vi "Dashboard Main.vi"() -> ()   [LabVIEW 2012]
uses:
  <vilib>/event_ctls.llb/eventvkey.ctl
  <vilib>/Utility/config.llb/Read Key (String).vi
  <vilib>/Utility/config.llb/Read Key (I32).vi
  <vilib>/Utility/config.llb/Write Key (String).vi
  <vilib>/Utility/config.llb/Write Key (I32).vi
  <vilib>/Utility/config.llb/NI_LVConfig.lvlib
  <vilib>/vision/NI_Vision_Development_Module.lvlib
panel:
  out "Battery Value":dbl(slide) scale=0.0..14.0 scale format="%#_2e"
  out "Battery":sgl(graph)
  in  "Camera Settings":T1={"Frate Rate"=30, "Compression"=30, "Size"=1} {"Frate Rate" scale=1.0..30.0; "Size" items=["640x480", "320x240", "160x120"]}
  out "Mode":T2(ring)=enum."Auto Disabled"
  out "Camera IP":string
  out "JS1 Z":dbl(slide) scale=-1.0..1.0 scale format="%#_2e"
  out "JS2 Z":dbl(slide) scale=-1.0..1.0 scale format="%#_2e"
  out "Joystick 1":cluster{"X":dbl, "Y":dbl}[](graph)
  out "Joystick 2":cluster{"X":dbl, "Y":dbl}[](graph)
  out "JS Buttons 1":T3
  out "JS Buttons 2":T3
  out "MotorSlide4":dbl(slide) scale=-1.0..1.0 scale format="%#_2e"
  out "MotorSlide3":dbl(slide) scale=-1.0..1.0 scale format="%#_2e"
  out "MotorSlide2":dbl(slide) scale=-1.0..1.0 scale format="%#_2e"
  in  "MotorName3":string="Front Left"
  in  "MotorName4":string="Front Right"
  in  "MotorName1":string="Rear Left"
  in  "MotorName2":string="Rear Right"
  out "MotorChart4":dbl(graph)
  out "MotorChart3":dbl(graph)
  out "MotorChart2":dbl(graph)
  out "MotorSlide1":dbl(slide) scale=-1.0..1.0 scale format="%#_2e"
  out "MotorChart1":dbl(graph)
  out "Robot IP":string
  in  "Dashboard Tab":enum32{"Operation", "Test", "Checklist"}(tab)
  in  "Checkbox 2":bool
  in  "Checkbox 1":bool
  in  "Slider 1":dbl(slide) scale=0.0..100.0
  out "Target Center":dbl[](array[numeric])
  in  "Slider":dbl(slide) scale=0.0..100.0 scale format="%#_3g"
  in  "On/Off":bool caption="Solenoid"
  in  "Test Name":u16(ring) items=["Select the test to run...", "Example Test", "-------------------------------", "List of tests is built in robot code.", "Replace with your own automated tests."]
  in  "Test Tree":string(tree)
  in  "Motor":cluster{"Value":dbl, "Enable":bool} {"Value" scale=-1.0..1.0 scale format="%#_3g"}
  out "Progress":T4 {"Test Progress" scale=0.0..100.0}
  in  "Rev/Fwd":cluster{"Forward":bool, "Reverse":bool}
  in  "Ring":u16(ring) items=["Auto", "Fixed indoor", "Fixed outdoor 1", "Fixed outdoor 2", "Fixed fluorescent 1", "Fixed fluorescent 2", "Hold current"]
  in  "Listbox":i32(listbox)
  in  "Viewer":T5(tab)
  out "Mbps":dbl format="%#.1g"
  in  "Enable":bool
  in  "DB Camera Config":bool
  out "Mbps":bool
  out "fps":dbl format="%#.1g"
  out "Image Error Message":string="Timeout in Camera Communications"
  out "Camera Image":T6(plugin-control)
  out "Buttons 1":cluster{"1":bool, "2":bool, "3":bool}
  out "Kinect 1":cluster{"X":dbl, "Y":dbl, "Z":dbl} {"X" scale=1.0..-1.0; "Y" scale=1.0..-1.0; "Z" scale=1.0..-1.0}
  out "Buttons 2":cluster{"1":bool, "2":bool, "3":bool}
  out "Kinect 2":cluster{"X":dbl, "Y":dbl, "Z":dbl} {"X" scale=1.0..-1.0; "Y" scale=1.0..-1.0; "Z" scale=1.0..-1.0}
  out "Version":string
  out "Skeleton Picture":picture
  out "Players":i8
  out "Tree":string(tree)
  out "Camera Image 2":T6(plugin-control)
  in  "Hue Range":cluster{dbl, dbl}
  in  "Sat Range":cluster{dbl, dbl}
  in  "Lum Range":cluster{dbl, dbl}
  # "Drive & Motors"
  # "Robot IP:"
  # "Customize by placing controls and indicators here and name to match\nDashboard Variables on robot."
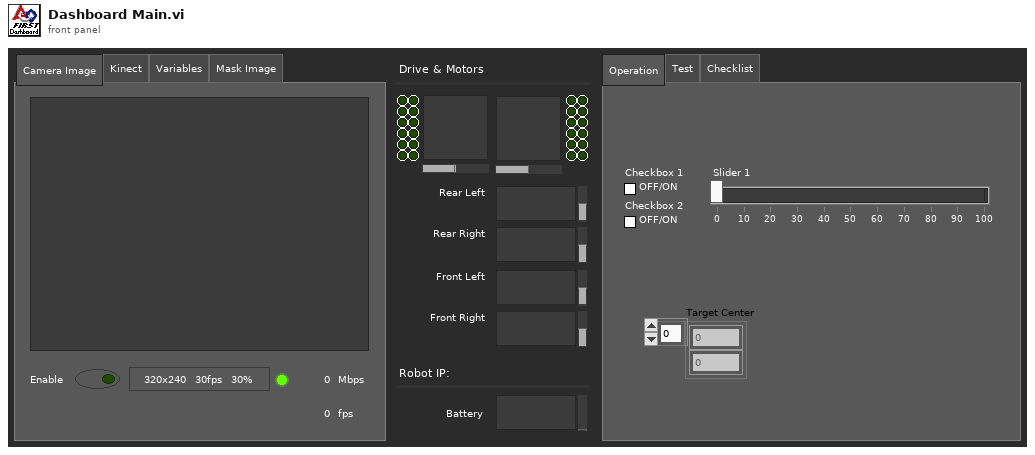
[diagram p1: front panel]
types:
  T1 = cluster{"Frate Rate":i32, "Compression":i32, "Size":u16}
  T2 = enum8{"Tele-Op Disabled", "Tele-Op Enabled", "Auto Disabled", "Auto Enabled", "Test Disabled", "Test Enabled", ""}
  T3 = cluster{bool, bool, bool, bool, bool, bool, bool, bool, bool, bool, bool, bool}
  T4 = cluster{"Test Progress":u8, "Test Progress Text":string}
  T5 = enum32{"Camera Image", "Kinect", "Variables", "Mask Image"}
  T6 = typedef "IMAQ Image.ctl" = refnum<image>
  T7 = typedef "Image Type" = u32
  T8 = typedef "LVBoundsTypeDef.ctl" = cluster{"Width":u32, "Height":u32}
  T9 = typedef "SkeletonTrackState.ctl" = enum32{"NotTracked", "PositionOnly", "Tracked"}
  T10 = cluster{"TrackingState":u8[], "Position":cluster{"x":sgl, "y":sgl, "z":sgl}, cluster{"x":sgl, "y":sgl, "z":sgl, sgl}[], "TrackState":T9}
  T11 = cluster{cluster{"ScaledToPercentRange":dbl, "ScaledToPercentRange":dbl, "ScaledToPercentRange":dbl}, cluster{bool, bool, bool}}[]
  T12 = cluster{cluster{"ScaledToPercentRange":dbl, "ScaledToPercentRange":dbl, "ScaledToPercentRange":dbl}, cluster{bool, bool, bool}}
  T13 = cluster{"ScaledToPercentRange":dbl, "ScaledToPercentRange":dbl, "ScaledToPercentRange":dbl}
  T14 = typedef "LVRectTypeDef.ctl" = cluster{"Left":i16, "Top":i16, "Right":i16, "Bottom":i16}
  T15 = cluster{"Competition mode":bool, "Robot Link":bool, "Autonomous":bool, "Enabled":bool, "E-Stop":bool, "Simulated":bool, "TestMode":bool, "Docked Window":bool}
  T16 = cluster{"Boolean Array[0]":bool, "Boolean Array[1]":bool, "Boolean Array[2]":bool, "Boolean Array[3]":bool, "Boolean Array[4]":bool, "Boolean Array[5]":bool, "Boolean Array[6]":bool, "Boolean Array[7]":bool, "Boolean Array[8]":bool, "Boolean Array[9]":bool, "Boolean Array[10]":bool, "Boolean Array[11]":bool}
  T17 = cluster{"Position":cluster{"X":dbl, "Y":dbl}, "Distance (ft)":dbl, "Center":bool}[]
  T18 = cluster{"Rect Coverage":i32, "X Edge Strength":i32, "Y Edge Strength":i32, "Center":i32, "Outer":i32}
  T19 = cluster{cluster{"Left":dbl, "Top":dbl, "Right":dbl, "Bottom":dbl}, "Scores":dbl[], cluster{"Long":dbl, "Short":dbl}}[]
  T20 = cluster{"Target Center (-1 to 1)":cluster{"X":dbl, "Y":dbl}, "Distance (ft)":dbl, "Center Target":bool}
  T21 = cluster{"Target Center (-1 to 1)":cluster{"X":dbl, "Y":dbl}, "Distance (ft)":dbl, "Center Target":bool}[]
  T22 = cluster{"Left":dbl, "Top":dbl, "Right":dbl, "Bottom":dbl}
  T23 = typedef "NI_LVConfig.lvlib/Config Data RefNum.ctl" = refnum<k1>
  T24 = typedef "eventvkey.ctl" = enum16{"ASCII", "Enter", "Return", "Shift", "Ctrl", "Alt", "Cmd", "Opt", "Caps", "NumLock", "Clear", "Break", "Up", "Down", "Left", "Right", "Insert", "Delete", "Home", "End", "PageUp", "PageDown", "Escape", "Help", "Pause", "ScrollLock", "F1", "F2", "F3", "F4", "F5", "F6", "F7", "F8", "F9", "F10", "F11", "F12", "F13", "F14", "F15", "F16", "F17", "F18", "F19", "F20", "F21", "F22", "F23", "F24", "Play", "VolumeUp", "VolumeDown", "Mute", "Two Byte Char"}
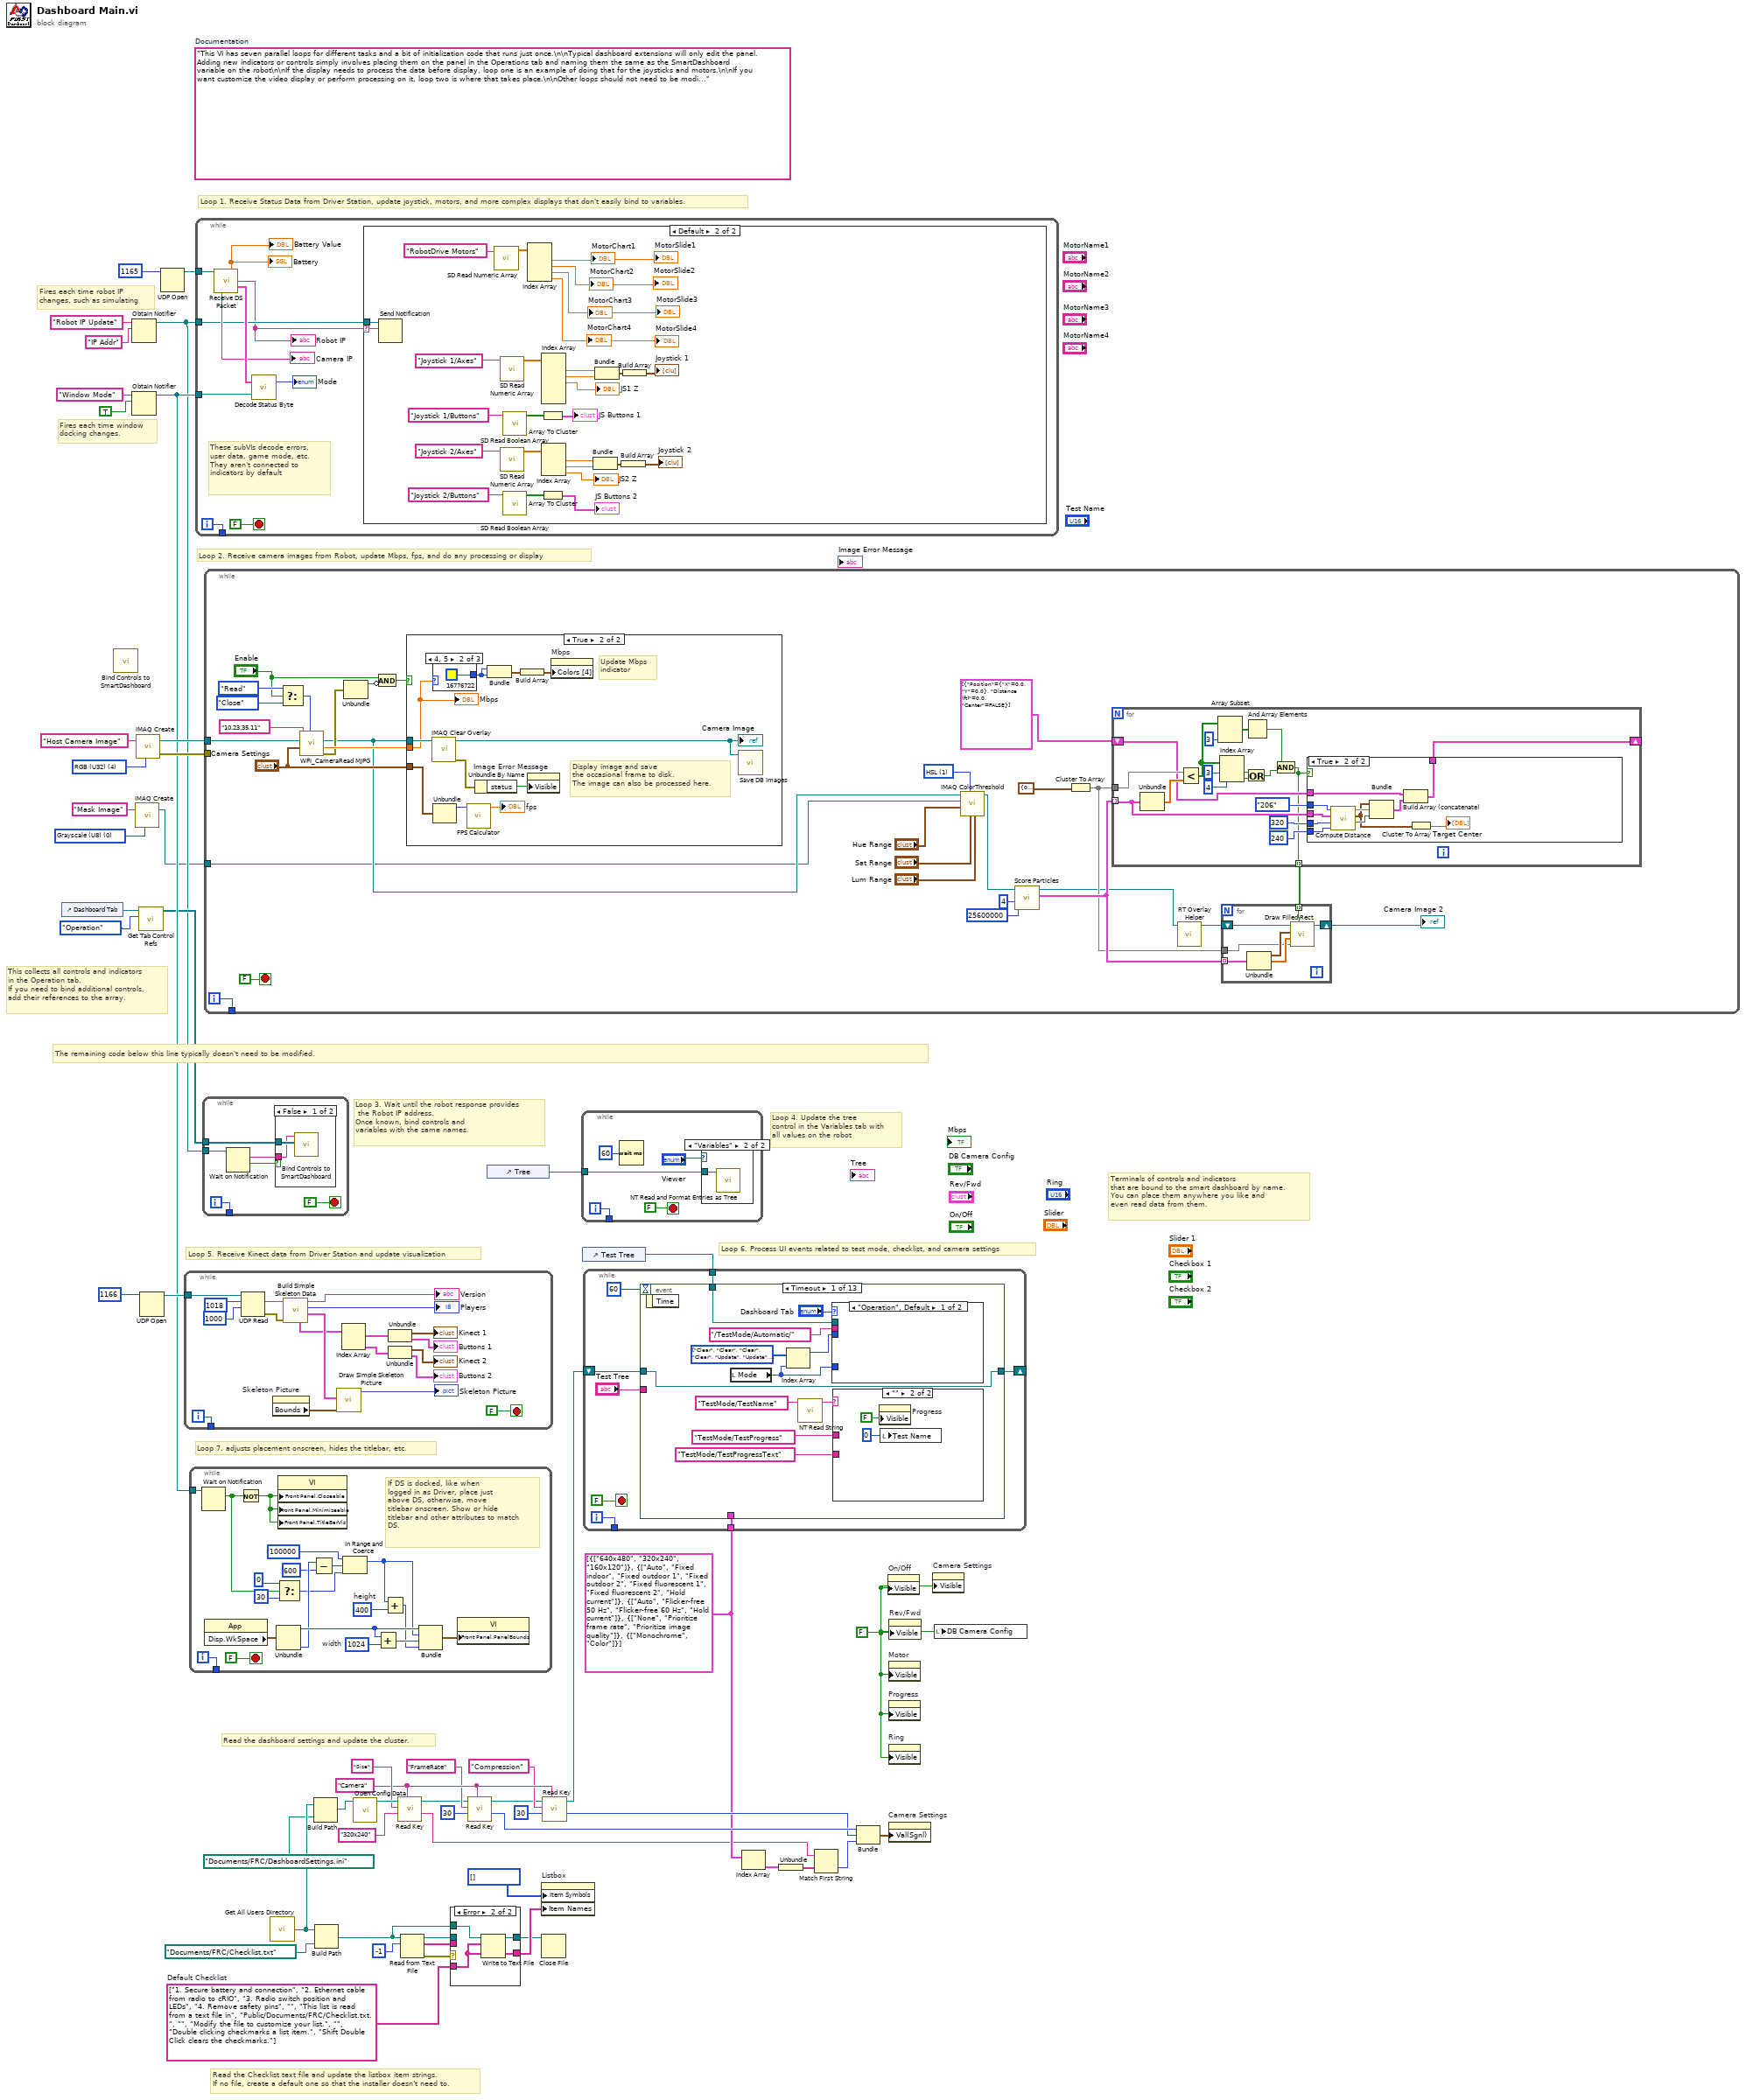
[diagram p0: block diagram]
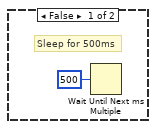
[diagram p4: hidden frame]
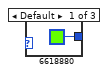
[diagram p5: hidden frame]
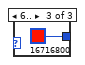
[diagram p6: hidden frame]
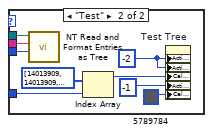
[diagram p8: hidden frame]
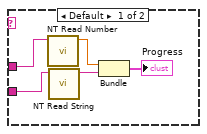
[diagram p9: hidden frame]
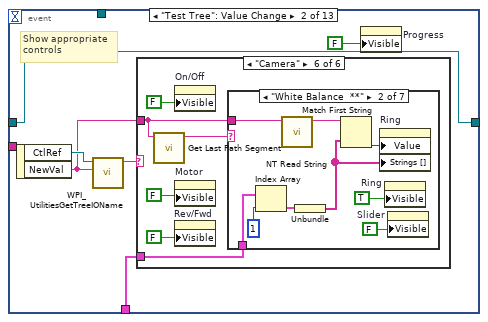
[diagram p10: hidden frame]
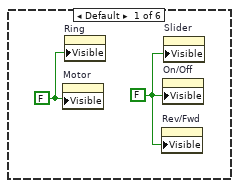
[diagram p11: hidden frame]
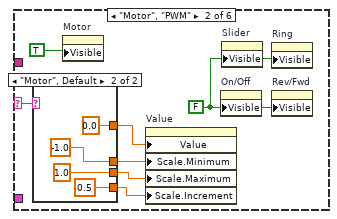
[diagram p12: hidden frame]
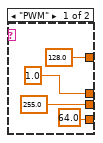
[diagram p13: hidden frame]
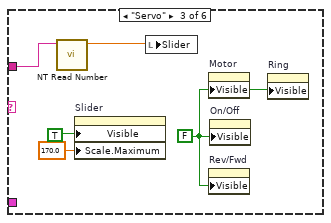
[diagram p14: hidden frame]
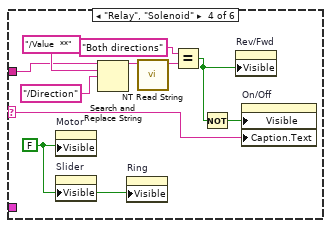
[diagram p15: hidden frame]
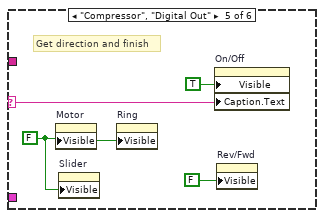
[diagram p16: hidden frame]
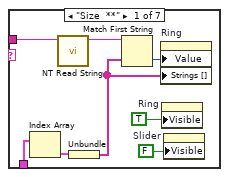
[diagram p17: hidden frame]
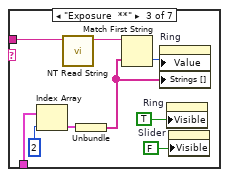
[diagram p18: hidden frame]
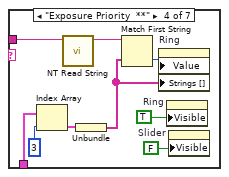
[diagram p19: hidden frame]
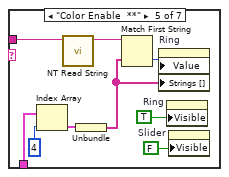
[diagram p20: hidden frame]
diagram:
  w3 = T7 0 items=["Grayscale (U8)", "Grayscale (I16)", "Grayscale (SGL)", "Complex (CSG)", "RGB (U32)", "HSL (U32)", "RGB (U64)"] ("Image Type")
  w26 = "Camera"
  w18 = cluster{string[]}[] [{["640x480", "320x240", "160x120"]}, {["Auto", "Fixed indoor", "Fixed outdoor 1", "Fixed outdoor 2", "Fixed fluorescent 1", "Fixed fluorescent 2", "Hold current"]}, {["Auto", "Flicker-free 50 Hz", "Flicker-free 60 Hz", "Hold current"]}, {["None", "Prioritize frame rate", "Prioritize image quality"]}, {["Monochrome", "Color"]}]
  w34 = string[] ["1. Secure battery and connection", "2. Ethernet cable from radio to cRIO", "3. Radio switch position and LEDs", "4. Remove safety pins", "", "This list is read from a text file in", "Public/Documents/FRC/Checklist.txt.", "", "Modify the file to customize your list.", "", "Double clicking checkmarks a list item.", "Shift Double Click clears the checkmarks."]  # Default Checklist
  w32 = FALSE ("Visible")
  (unwired) "This VI has seven parallel loops for different tasks and a bit of initialization code that runs just once.\n\nTypical dashboard extensions will only edit the panel. Adding new indicators or controls simply involves placing them on the panel in the Operations tab and naming them the same as the SmartDashboard variable on the robot\n\nIf the display needs to process the data before display, loop one is an example of doing that for the joysticks and motors.\n\nIf you want customize the video display or perform processing on it, loop two is where that takes place.\n\nOther loops should not need to be modified. They are pretty standard, and document the task they perform."  # Documentation
  w53 = T7 4 items=["Grayscale (U8)", "Grayscale (I16)", "Grayscale (SGL)", "Complex (CSG)", "RGB (U32)", "HSL (U32)", "RGB (U64)"] ("Image Type")
  # "Fires each time robot IP\nchanges, such as simulating"
  # "Fires each time window\ndocking changes."
  # "Read the Checklist text file and update the listbox item strings.\nIf no file, create a default one so that the installer doesn't need to."
  # "This collects all controls and indicators\nin the Operation tab.\nIf you need to bind additional controls,\nadd their references to the array."
  # "The remaining code below this line typically doesn't need to be modified."
  # "Loop 6. Process UI events related to test mode, checklist, and camera settings"
  # "Read the dashboard settings and update the cluster."
  # "Terminals of controls and indicators\nthat are bound to the smart dashboard by name.\nYou can place them anywhere you like and\neven read data from them."
  # "Loop 4. Update the tree\ncontrol in the Variables tab with\nall values on the robot"
  # "Loop 3. Wait until the robot response provides\n the Robot IP address.\nOnce known, bind controls and\nvariables with the same names."
  # "Loop 5. Receive Kinect data from Driver Station and update visualization"
  # "Loop 7. adjusts placement onscreen, hides the titlebar, etc."
  # "Loop 1. Receive Status Data from Driver Station, update joystick, motors, and more complex displays that don't easily bind to variables."
  # "Loop 2. Receive camera images from Robot, update Mbps, fps, and do any processing or display"
  n1 = control-ref of="Dashboard Tab"() -> (w47:refnum<vi>)
  n2 = call <vilib>:"Bind Controls to SmartDashboard.vi"() -> ()  [unwired: 12 in]
  n3 = Obtain Notifier(name (unnamed)="Robot IP Update", notification data type="IP Addr" ("name (unnamed)")) -> (notifier out=w4:refnum<notifier>)  [unwired: 2 in, 2 out]
  n4 = Obtain Notifier(name (unnamed)="Window Mode", notification data type=TRUE) -> (notifier out=w38:refnum<notifier>)  [unwired: 2 in, 2 out]
  n5 = call "IMAQ Create"("Image Name"="Mask Image", "Image Type"=w3) -> ("New Image"=w1:T6)  [unwired: 2 in, 2 out]
  n6 = call "IMAQ Create"("Image Name"="Host Camera Image", "Image Type"=w53) -> ("New Image"=w51:T6, "error out"=w50:errorcluster)  [unwired: 2 in, 1 out]
  n7 = call <vilib>:"Get Tab Control Refs.vi"("Page Index"=enum32{"Operation", "Test"}."Operation" ("Dashboard Tab"), "TabControl in"=w47) -> ("ControlsOnPage"=w5:refnum<vi>[])  [unwired: 9 in]
  n8 = UDP Open(11:u16 1166 ("port")) -> (port=w48:refnum<k16>)  [unwired: 2 in, 4 out]
  n9 = UDP Open(11:u16 1165 ("port")) -> (port=w54:refnum<k16>)  [unwired: 2 in, 4 out]
  n10 = while {
    tunnel: w48 -> [w72]
    tunnel: [w57] -> _
    i -> [w57]
    stop <- FALSE stop-if-true
    n11 = UDP Read(connection ID=w72, max size (548)=1018 ("bytes to read"), timeout ms (25000)=1000) -> (data out=w66:string, error out=w56:errorcluster)  [unwired: 1 in, 3 out]
    n12 = property on="Skeleton Picture" class="Pict"() -> ("Bounds"=w68:T8)  [unwired: 2 in, 2 out]
    n13 = call "Build Simple Skeleton Data.vi"("error in (no error)"=w56, "data in"=w66) -> ("Skeleton Data"=w67:T10, "NumPlayers"=→"Players":i8, "Version String"=→"Version":string, "Simple Joystick Info"=w64:T11)  [unwired: 5 in, 1 out]
    n14 = call "Draw Simple Skeleton Picture.vi"("Bounds"=w68, "Simple Skeleton"=w67) -> ("new picture out"=→"Skeleton Picture":picture)  [unwired: 9 in]
    n15 = Index Array(array=w64) -> (element #1=w63:T12, element #2=w62:T12)  [unwired: 2 in]
    n16 = Unbundle(w63) -> (→"Kinect 1":T13, →"Buttons 1":cluster{bool, bool, bool})
    n17 = Unbundle(w62) -> (→"Kinect 2":T13, →"Buttons 2":cluster{bool, bool, bool})
  }
  n18 = while {
    tunnel: w38 -> [w93]
    tunnel: [w91] -> _
    i -> [w91]
    stop <- FALSE stop-if-true
    w83 = 1024  # width
    w86 = 400  # height
    # "If DS is docked, like when\nlogged in as Driver, place just\nabove DS, otherwise, move\ntitlebar onscreen. Show or hide\ntitlebar and other attributes to match\nDS."
    n19 = Wait on Notification(notifier=w93) -> (notification=w78:bool)  [unwired: 3 in, 3 out]
    n20 = property class="App"() -> ("Disp.WkSpace"=w89:T14)  [unwired: 2 in, 2 out]
    n21 = Not(x=w78) -> (.not. x?=w92:bool)
    n22 = Unbundle(w89) -> ("Left"=w87:i16, "Bottom"=w84:i16)  [unwired: 2 out]
    n23 = Select(t=0, s=w78, f=30) -> (s? t:f=w77:i32)
    n24 = property class="VI"("Front Panel.Closeable"=w92, "Front Panel.Minimizeable"=w92, "Front Panel.TitleBarVis"=w92) -> ()  [unwired: 2 in, 2 out]
    n25 = Subtract(x=w84, y=600) -> (x-y=w81:i32)
    n26 = In Range and Coerce(upper limit=100000, x=w81, lower limit=w77) -> (coerced(x)=w75:i32)  [unwired: 1 out]
    n27 = Add(x=w87, y=w83) -> (x+y=w88:i32)
    n28 = Add(x=w75, y=w86) -> (x+y=w85:i32)
    n29 = Bundle("Left"=w87, w75, w88, w85) -> (w90:cluster{"Left":i16, i32, i32, i32})  [unwired: 1 out]
    n30 = property class="VI"("Front Panel.PanelBounds"=w90) -> ()  [unwired: 2 in, 2 out]
  }
  n31 = while {
    tunnel: w54 -> [w102]
    tunnel: w4 -> [w96]
    tunnel: w38 -> [w100]
    tunnel: [w97] -> _
    i -> [w97]
    stop <- FALSE stop-if-true
    # "These subVIs decode errors, user data, game mode, etc.\nThey aren't connected to indicators by default"
    n32 = call "Receive DS Packet.vi"("Recv Socket"=w102) -> ("Battery"=→"Battery" →"Battery Value":sgl, "Robot IP Address"=w95:string, "Status"=w103:T15, "Camera IP Address"=→"Camera IP":string)  [unwired: 1 in, 10 out]
    "Robot IP" <- w95
    n33 = call "Decode Status Byte.vi"("Window Mode Notifier"=w100, "Status"=w103) -> ("Mode"=→"Mode":T2)  [unwired: 1 out]
    n34 = case shown="Default" w95 {
      selector: w95 -> [_ w105]
      tunnel: w96 -> [_ w106]
      frame "0.0.0.0" {
        # "Robot not responding, don't poll the variables"
      }
      frame Default {
        n35 = Send Notification(notification=w105, notifier=w106) -> ()  [unwired: 1 in, 2 out]
        n36 = call <vilib>:"SD Read Numeric Array.vi"("Name"="RobotDrive Motors") -> ("Numeric Array"=w129:dbl[])  [unwired: 8 in, 2 out]
        n37 = call <vilib>:"SD Read Numeric Array.vi"("Name"="Joystick 1/Axes") -> ("Numeric Array"=w122:dbl[])  [unwired: 8 in, 2 out]
        n38 = call <vilib>:"SD Read Numeric Array.vi"("Name"="Joystick 2/Axes") -> ("Numeric Array"=w116:dbl[])  [unwired: 8 in, 2 out]
        n39 = call <vilib>:"SD Read Boolean Array.vi"("Name"="Joystick 1/Buttons") -> ("Boolean Array"=w124:bool[])  [unwired: 8 in, 2 out]
        n40 = call <vilib>:"SD Read Boolean Array.vi"("Name"="Joystick 2/Buttons") -> ("Boolean Array"=w115:bool[])  [unwired: 8 in, 2 out]
        n41 = Index Array(array=w129) -> (element #1=→"MotorChart1" →"MotorSlide1":dbl, element #2=→"MotorSlide2" →"MotorChart2":dbl, element #3=→"MotorChart3" →"MotorSlide3":dbl, element #4=→"MotorChart4" →"MotorSlide4":dbl)  [unwired: 4 in]
        n42 = Array To Cluster(array=w124) -> (cluster=→"JS Buttons 1":T16)
        n43 = Array To Cluster(array=w115) -> (cluster=→"JS Buttons 2":T16)
        n44 = Index Array(array=w122) -> (element #1=w119:dbl, element #2=w120:dbl, element #3=→"JS1 Z":dbl)  [unwired: 6 in, 3 out]
        n45 = Index Array(array=w116) -> (element #1=w111:dbl, element #2=w110:dbl, element #3=→"JS2 Z":dbl)  [unwired: 3 in]
        n46 = Bundle("Numeric"=w111, "Numeric"=w110) -> (w112:cluster{"Numeric":dbl, "Numeric":dbl})  [unwired: 1 in]
        n47 = Bundle("Numeric"=w119, "Numeric"=w120) -> (w118:cluster{"Numeric":dbl, "Numeric":dbl})  [unwired: 1 in]
        n48 = Build Array(w112) -> (→"Joystick 2":cluster{"Numeric":dbl, "Numeric":dbl}[])
        n49 = Build Array(w118) -> (→"Joystick 1":cluster{"Numeric":dbl, "Numeric":dbl}[])
      }
    }
  }
  n50 = while {
    tunnel: w5 -> [w138]
    tunnel: w4 -> [w135]
    tunnel: [w133] -> _
    i -> [w133]
    stop <- FALSE stop-if-true
    n51 = Wait on Notification(notifier=w135) -> (notification=w134:string, timed out?=w136:bool)  [unwired: 3 in, 2 out]
    n52 = case shown="False" w136 {
      tunnel: w138 -> [w140 _]
      tunnel: w134 -> [w139 _]
      frame False {
        n53 = call <vilib>:"Bind Controls to SmartDashboard.vi"("Bound Control Refs"=w140, "Server IP Address"=w139) -> ()  [unwired: 10 in]
      }
      frame True {
      }
    }
  }
  n54 = while {
    tunnel: w51 -> [w167]
    tunnel: w50 -> [_]
    tunnel: [w169] -> _
    tunnel: w1 -> [w146]
    i -> [w169]
    stop <- FALSE stop-if-true
    w157 = u16 1 items=["RGB", "HSL", "HSV", "HSI"] ("Color Mode")
    n55 = Select(t=enum16{"Read", "Reopen", "Close"}."Read" ("Operation"), s="Enable", f=enum16{"Read", "Reopen", "Close"}."Close" ("Operation")) -> (s? t:f=w163:enum16{"Read", "Reopen", "Close"})
    n56 = call <vilib>:"WPI_CameraRead MJPG.vi"("Operation"=w163, "Camera Settings"="Camera Settings", "Image"=w167, "address"="10.23.35.11") -> ("error out"=w162:errorcluster, "Bandwidth (kbps)"=w166:dbl, "Image Out"=w147:T6)  [unwired: 5 in]
    n57 = Unbundle(w162) -> ("status"=w160:bool)  [unwired: 2 out]
    n58 = Compound Arithmetic op=AND("Enable", invert w160) -> (w159:bool)
    n59 = case shown="True" w159 {
      tunnel: "Camera Settings" -> [_ w210]
      tunnel: w147 -> [_ w213]
      tunnel: w166 -> [_ w212]
      frame False {
        # "Sleep for 500ms"
        n60 = Wait Until Next ms Multiple(millisecond multiple=u32 500) -> ()  [unwired: 1 out]
      }
      frame True {
        # "Display image and save\nthe occasional frame to disk.\nThe image can also be processed here."
        # "Update Mbps\nindicator"
        n61 = call "IMAQ Clear Overlay"("Image"=w213) -> ("error out"=w218:errorcluster, "Image Out"=w217:T6)  [unwired: 2 in, 7 out]
        "Camera Image" <- w217
        n62 = case shown="4, 5" w212 {
          tunnel: [u32 6618880 ("Color Box") u32 16776722 ("Color Box") u32 16716800 ("Color Box")] -> w214
          frame Default {
          }
          frame 4, 5 {
          }
          frame 6.. {
          }
        }
        n63 = Unbundle(w210) -> ("Frate Rate"=w209:i32)  [unwired: 2 out]
        n64 = call "FPS Calculator.vi"("Average Count"=w209) -> ("fps"=→"fps":dbl)  [unwired: 10 in]
        n65 = Unbundle By Name(w218) -> ("status"=w219:bool)
        n66 = Bundle("Color Box"=w214, "Color Box"=w214) -> (w216:cluster{"Color Box":u32, "Color Box":u32})  [unwired: 1 out]
        n67 = Build Array(w216) -> (w215:cluster{"Color Box":u32, "Color Box":u32}[])
        n68 = property on="Image Error Message" class="Str"("Visible"=w219) -> ()  [unwired: 2 in, 2 out]
        n69 = property on="Mbps" class="Bool (strict)"("Colors [4]"=w215) -> ()  [unwired: 2 in, 2 out]
        n70 = call "Save DB Images.vi"("Image"=w217) -> ()  [unwired: 2 in, 1 out]
        "Mbps" <- w212
      }
    }
    n71 = call "IMAQ ColorThreshold"("Blue or Luma or Val or Inten Range"="Lum Range", "Green or Sat Range"="Sat Range", "Color Mode"=w157, "Red or Hue Range"="Hue Range", "Image Dst"=w146, "Image Src"=w147) -> ("Image Dst Out"=w148:T6)  [unwired: 4 in, 1 out]
    n72 = call "Score Particles.vi"("Area Size Limit"=25600000, "Particle Count Limit"=4, "Image Refnum in"=w148) -> ("Scored Particle Info"=w151:T19, "Image Refnum out"=w149:T6)  [unwired: 7 in]
    n73 = Cluster To Array(cluster=T18 {"Rect Coverage"=0, "X Edge Strength"=0, "Y Edge Strength"=0, "Center"=0, "Outer"=0}) -> (array=w150:i32[])
    n74 = for {
      tunnel: w151 -> [w184] mode=indexing
      shift-right: [w179] -> _
      shift-left: T17 [{"Position"={"X"=0.0, "Y"=0.0}, "Distance (ft)"=0.0, "Center"=FALSE}] -> [w180]
      tunnel: w150 -> [w194]
      tunnel: [w178] -> w152 mode=indexing
      n75 = Unbundle(w184) -> ("Scores"=w195:dbl[])  [unwired: 2 out]
      n76 = Less?(x=w194, y=w195) -> (x < y?=w192:bool[])
      n77 = Array Subset(array=w192, length=3) -> (w189:bool[])  [unwired: 1 in]
      n78 = Index Array(array=w192, index #1=3 ("index"), index #2=4 ("index")) -> (element #1=w187:bool, element #2=w188:bool)
      n79 = Or(x=w187, y=w188) -> (x .or. y?=w186:bool)
      n80 = And Array Elements(Boolean array=w189) -> (logical AND=w185:bool)
      n81 = And(x=w185, y=w186) -> (x .and. y?=w178:bool)
      n82 = case shown="True" w178 {
        tunnel: w184 -> [_ w207]
        tunnel: enum16{"206", "1011"}."206" ("Camera Type") -> [_ w206]
        tunnel: 320 ("X Image Resolution") -> [_ w205]
        tunnel: 240 ("Y Image Resolution") -> [_ w204]
        tunnel: w180 -> [w196 w200]
        tunnel: [w196 w199] -> w179
        frame False {
        }
        frame True {
          n83 = call "Compute Distance.vi"("Y Image Resolution"=w204, "X Image Resolution"=w205, "Particle Scores"=w207, "Camera Type"=w206) -> ("Center Target"=w202:bool, "Target Center (-1 to 1)"=w198:cluster{"X":dbl, "Y":dbl}, "Distance (ft)"=w203:dbl)  [unwired: 5 in]
          n84 = Bundle("Target Center (-1 to 1)"=w198, "Distance (ft)"=w203, "Center Target"=w202) -> (w201:T20)  [unwired: 1 in]
          n85 = Build Array (concatenate)(w200, w201) -> (w199:T21)
          n86 = Cluster To Array(cluster=w198) -> (array=→"Target Center":dbl[])
        }
      }
    }
    n87 = call "RT Overlay Helper.vi"("Refnum in"=w149) -> ("Refnum out"=w153:T6)  [unwired: 10 in]
    n88 = for {
      shift-right: [w176] -> w144
      shift-left: w153 -> [w177]
      tunnel: w151 -> [w173] mode=indexing
      tunnel: w150 -> [w172]
      tunnel: w152 -> [w171] mode=indexing
      n89 = Unbundle(w173) -> (w174:T22, "Scores"=w175:dbl[])  [unwired: 1 out]
      n90 = call "Draw Filled Rect.vi"("Limit Passed"=w171, "Limits"=w172, "Scores"=w175, "Bounding Box"=w174, "image in"=w177) -> ("image out"=w176:T6)  [unwired: 6 in]
    }
    "Camera Image 2" <- w144
  }
  n91 = call "Get All Users Directory.vi"() -> ("All User Path"=w31:path)
  n92 = Build Path(base path=w31, name or relative path=path "Documents/FRC/DashboardSettings.ini") -> (appended path=w30:path)
  n93 = Build Path(base path=w31, name or relative path=path "Documents/FRC/Checklist.txt") -> (appended path=w35:path)
  n94 = call <vilib>:"Open Config Data.vi"("configuration file path"=w30) -> ("refnum"=w29:T23)  [unwired: 8 in, 2 out]
  n95 = call-poly <vilib>:"Read Key.vi"("section"=w26, "default value"="320x240", "key"="Size", "refnum"=w29) -> ("value"=w16:string, "refnum out"=w11:T23)  [unwired: 2 in, 4 out]
  n96 = Read from Text File(file (use dialog)=w35, count=-1 ("timeout ms (25000)")) -> (refnum out=w13:refnum<file>, text=w36:string[], error out=w37:errorcluster)  [unwired: 2 in, 1 out]
  n97 = case shown="Error" w37 {
    tunnel: w36 -> [w224 _]
    tunnel: [w224 w226] -> w33
    tunnel: w34 -> [_ w226]
    tunnel: w35 -> [_ w227]
    tunnel: [w223 w225] -> w12
    tunnel: w13 -> [w223 _]
    frame No Error {
    }
    frame Error {
      n98 = Write to Text File(file (use dialog)=w227, text=w226) -> (refnum out=w225:refnum<file>)  [unwired: 2 in, 2 out]
    }
  }
  n99 = call-poly <vilib>:"Read Key.vi"("section"=w26, "default value"=30, "key"="FrameRate", "refnum"=w11) -> ("value"=w21:i32, "refnum out"=w10:T23)  [unwired: 1 in, 5 out]
  n100 = control-ref of="Tree"() -> (w6:refnum<vi>)
  n101 = property on="Listbox" class="LstBox (strict)"("Item Symbols"=i32[] [], "Item Names"=w33) -> ()  [unwired: 2 in, 2 out]
  n102 = Close File(refnum=w12) -> ()  [unwired: 1 in, 2 out]
  n103 = call-poly <vilib>:"Read Key.vi"("section"=w26, "default value"=30, "key"="Compression", "refnum"=w10) -> ("value"=w20:i32, "refnum out"=w8:T23)  [unwired: 1 in, 5 out]
  n104 = while {
    tunnel: [w229] -> _
    tunnel: w6 -> [w228]
    i -> [w229]
    stop <- FALSE stop-if-true
    n105 = Wait (ms)(milliseconds to wait=u32 60) -> ()  [unwired: 1 out]
    n106 = case shown="\"Variables\"" "Viewer" {
      tunnel: w228 -> [_ w233]
      frame Default {
      }
      frame "Variables" {
        n107 = call <vilib>:"NT Read and Format Entries as Tree.vi"("Tree Refnum"=w233) -> ()  [unwired: 9 in, 2 out]
      }
    }
  }
  n108 = control-ref of="Test Tree"() -> (w7:refnum<vi>)
  n109 = while {
    tunnel: w18 -> [w238]
    shift-right: [w237] -> _
    shift-left: w8 -> [w236]
    tunnel: [w235] -> _
    tunnel: w7 -> [w234]
    i -> [w235]
    stop <- FALSE stop-if-true
    n110 = event shown="[0] Timeout" {
      selector: _ -> [_ _ _ _ _ _ _ _ _ _ _ _ _]
      dyn-events: _ -> [_ _ _ _ _ _ _ _ _ _ _ _ _]
      timeout: u32 60 ("milliseconds to wait") -> [_ _ _ _ _ _ _ _ _ _ _ _ _]
      tunnel: w234 -> [w248 _ _ _ _ _ _ _ _ _ _ _ _]
      tunnel: "Test Tree" -> [_ _ _ _ _ _ _ _ w442 w450 w452 w456 w464]
      tunnel: w238 -> [_ w270 _ _ _ _ w406 w436 _ _ _ _ _]
      tunnel: [w242 w269 _ w372 w380 w392 w405 w429 w441 w448 w451 w455 w463] -> w237
      tunnel: w236 -> [w242 w269 _ w372 w380 w392 w404 w429 w441 w448 w451 w455 w463]
      event Timeout {
        w247 = enum16{"Update", "Clear"}[] [enum."Clear", enum."Clear", enum."Clear", enum."Clear", enum."Update", enum."Update", enum."Clear"] items=["Update", "Clear"]
        n111 = event-data() -> ()  [unwired: 1 in, 1 out]
        n112 = local read "Mode"() -> (w245:T2)
        n113 = Index Array(array=w247, index=w245) -> (element=w246:enum16{"Update", "Clear"})
        n114 = call <vilib>:"NT Read String.vi"("Name"="TestMode/TestName") -> ("String"=w251:string)  [unwired: 9 in, 1 out]
        n115 = case shown="\"Operation\", Default" "Dashboard Tab" {
          tunnel: w248 -> [_ w261]
          tunnel: "/TestMode/Automatic/" ("Name Pattern") -> [_ w260]
          tunnel: w246 -> [_ w259]
          tunnel: w245 -> [_ w257]
          frame "Operation", Default {
          }
          frame "Test" {
            w256 = -2 ("Active Item:Row Number")
            n116 = call <vilib>:"NT Read and Format Entries as Tree.vi"("Operation"=w259, "Name Pattern"=w260, "Tree Refnum"=w261) -> ()  [unwired: 7 in, 2 out]
            n117 = Index Array(array=u32[] [14013909, 14013909, 14013909, 14013909, 14013909, 16777215, 14013909], index=w257) -> (element=w255:u32)
            n118 = property on="Test Tree" class="Tree (strict)"("Active Item Row Number"=w256, "ActiveColNum"=w256, "CellBG"=w255, "Active Item Row Number"=-1 ("Active Item:Row Number"), "CellBG"=u32 5789784 ("Color Box")) -> ()  [unwired: 2 in, 2 out]
          }
        }
        n119 = case shown="\"\"" w251 {
          tunnel: "TestMode/TestProgress" ("Name") -> [w263 _]
          tunnel: "TestMode/TestProgressText" ("Name") -> [w262 _]
          frame Default {
            n120 = call <vilib>:"NT Read Number.vi"("Name"=w263) -> ("Numeric"=w264:dbl)  [unwired: 9 in, 1 out]
            n121 = call <vilib>:"NT Read String.vi"("Name"=w262) -> ("String"=w265:string)  [unwired: 9 in, 1 out]
            n122 = Bundle("Numeric"=w264, "String"=w265) -> (→"Progress":cluster{"Numeric":dbl, "String":string})  [unwired: 1 in]
          }
          frame "" {
            n123 = property on="Progress" class="Clust (strict)"("Visible"=FALSE) -> ()  [unwired: 2 in, 2 out]
            n124 = local write "Test Name"(u16 0) -> ()
          }
        }
      }
      event "Test Tree": Value Change {
        # "Show appropriate\ncontrols"
        n125 = event-data() -> ("CtlRef"=w273:refnum<vi>, "NewVal"=w271:string)  [unwired: 1 in]
        n126 = call <vilib>:"WPI_UtilitiesGetTreeIOName.vi"("NewVal"=w271, "TreeControl in"=w273) -> ("I/O Name"=w274:string)  [unwired: 9 in]
        n127 = case shown="\"Camera\"" w274 {
          selector: w274 -> [_ w281 _ w299 w308 _]
          tunnel: w271 -> [_ _ w296 w298 _ w315]
          tunnel: w270 -> [_ _ _ _ _ w314]
          frame Default {
            w276 = FALSE ("Visible")
            w275 = FALSE ("Visible")
            n128 = property on="Motor" class="Clust (strict)"("Visible"=w275) -> ()  [unwired: 2 in, 2 out]
            n129 = property on="Ring" class="Ring (strict)"("Visible"=w275) -> ()  [unwired: 2 in, 2 out]
            n130 = property on="Rev/Fwd" class="Clust (strict)"("Visible"=w276) -> ()  [unwired: 2 in, 2 out]
            n131 = property on="On/Off" class="Bool (strict)"("Visible"=w276) -> ()  [unwired: 2 in, 2 out]
            n132 = property on="Slider" class="Slide (strict)"("Visible"=w276) -> ()  [unwired: 2 in, 2 out]
          }
          frame "Motor", "PWM" {
            w282 = FALSE ("Visible")
            n133 = case shown="\"Motor\", Default" w281 {
              tunnel: [1.0 ("Value") -1.0 ("Value")] -> w280
              tunnel: [255.0 ("Value") 1.0 ("Value")] -> w279
              tunnel: [128.0 ("Value") 0.0 ("Value")] -> w278
              tunnel: [64.0 ("Value") 0.5 ("Value")] -> w277
              frame "PWM" {
              }
              frame "Motor", Default {
              }
            }
            n134 = property on="Motor" class="Clust (strict)"("Visible"=TRUE) -> ()  [unwired: 2 in, 2 out]
            n135 = property on="Value" class="Slide (strict)"("Value"=w278, "Scale.Minimum"=w280, "Scale.Maximum"=w279, "Scale.Increment"=w277) -> ()  [unwired: 2 in, 2 out]
            n136 = property on="On/Off" class="Bool (strict)"("Visible"=w282) -> ()  [unwired: 2 in, 2 out]
            n137 = property on="Slider" class="Slide (strict)"("Visible"=w282) -> ()  [unwired: 2 in, 2 out]
            n138 = property on="Ring" class="Ring (strict)"("Visible"=w282) -> ()  [unwired: 2 in, 2 out]
            n139 = property on="Rev/Fwd" class="Clust (strict)"("Visible"=w282) -> ()  [unwired: 2 in, 2 out]
          }
          frame "Servo" {
            w294 = FALSE ("Visible")
            n140 = call <vilib>:"NT Read Number.vi"("Name"=w296) -> ("Numeric"=w295:dbl)  [unwired: 9 in, 1 out]
            n141 = property on="Slider" class="Slide (strict)"("Visible"=TRUE, "Scale.Maximum"=170.0 ("Scale.Range:Maximum")) -> ()  [unwired: 2 in, 2 out]
            n142 = local write "Slider"(w295) -> ()
            n143 = property on="Motor" class="Clust (strict)"("Visible"=w294) -> ()  [unwired: 2 in, 2 out]
            n144 = property on="Rev/Fwd" class="Clust (strict)"("Visible"=w294) -> ()  [unwired: 2 in, 2 out]
            n145 = property on="On/Off" class="Bool (strict)"("Visible"=w294) -> ()  [unwired: 2 in, 2 out]
            n146 = property on="Ring" class="Ring (strict)"("Visible"=w294) -> ()  [unwired: 2 in, 2 out]
          }
          frame "Relay", "Solenoid" {
            w297 = FALSE ("Visible")
            n147 = property on="Motor" class="Clust (strict)"("Visible"=w297) -> ()  [unwired: 2 in, 2 out]
            n148 = property on="Slider" class="Slide (strict)"("Visible"=w297) -> ()  [unwired: 2 in, 2 out]
            n149 = Search and Replace String(input string=w298, search string="/Value  **", replace string="/Direction") -> (result string=w304:string)  [unwired: 5 in, 3 out]
            n150 = property on="Ring" class="Ring (strict)"("Visible"=w297) -> ()  [unwired: 2 in, 2 out]
            n151 = call <vilib>:"NT Read String.vi"("Name"=w304) -> ("String"=w302:string)  [unwired: 9 in, 1 out]
            n152 = Equal?(x="Both directions", y=w302) -> (x = y?=w300:bool)
            n153 = Not(x=w300) -> (.not. x?=w301:bool)
            n154 = property on="Rev/Fwd" class="Clust (strict)"("Visible"=w300) -> ()  [unwired: 2 in, 2 out]
            n155 = property on="On/Off" class="Bool (strict)"("Visible"=w301, "Caption.Text"=w299) -> ()  [unwired: 2 in, 2 out]
          }
          frame "Compressor", "Digital Out" {
            w307 = FALSE ("Visible")
            # "Get direction and finish"
            n156 = property on="Motor" class="Clust (strict)"("Visible"=w307) -> ()  [unwired: 2 in, 2 out]
            n157 = property on="Slider" class="Slide (strict)"("Visible"=w307) -> ()  [unwired: 2 in, 2 out]
            n158 = property on="Ring" class="Ring (strict)"("Visible"=w307) -> ()  [unwired: 2 in, 2 out]
            n159 = property on="On/Off" class="Bool (strict)"("Visible"=TRUE, "Caption.Text"=w308) -> ()  [unwired: 2 in, 2 out]
            n160 = property on="Rev/Fwd" class="Clust (strict)"("Visible"=FALSE) -> ()  [unwired: 2 in, 2 out]
          }
          frame "Camera" {
            n161 = call <vilib>:"Get Last Path Segment.vi"("String in"=w315) -> ("String out"=w316:string)  [unwired: 10 in]
            n162 = property on="On/Off" class="Bool (strict)"("Visible"=FALSE) -> ()  [unwired: 2 in, 2 out]
            n163 = property on="Motor" class="Clust (strict)"("Visible"=FALSE) -> ()  [unwired: 2 in, 2 out]
            n164 = property on="Rev/Fwd" class="Clust (strict)"("Visible"=FALSE) -> ()  [unwired: 2 in, 2 out]
            n165 = case shown="\"White Balance  **\"" w316 {
              tunnel: w315 -> [w322 w331 w340 w349 w358 _ w364]
              tunnel: w314 -> [w320 w328 w337 w346 w355 _ _]
              frame "Size  **" {
                n166 = Index Array(array=w320) -> (element=w319:cluster{string[]})  [unwired: 1 in]
                n167 = call <vilib>:"NT Read String.vi"("Name"=w322) -> ("String"=w321:string)  [unwired: 9 in, 1 out]
                n168 = Unbundle(w319) -> (w317:string[])
                n169 = Match First String(2:w317, 3:w321) -> (0:w318:i32)  [unwired: 1 out]
                n170 = property on="Ring" class="Ring (strict)"("Value"=w318, "Strings []"=w317) -> ()  [unwired: 2 in, 2 out]
                n171 = property on="Ring" class="Ring (strict)"("Visible"=TRUE) -> ()  [unwired: 2 in, 2 out]
                n172 = property on="Slider" class="Slide (strict)"("Visible"=FALSE) -> ()  [unwired: 2 in, 2 out]
              }
              frame "White Balance  **" {
                n173 = Index Array(array=w328, index=1) -> (element=w329:cluster{string[]})
                n174 = call <vilib>:"NT Read String.vi"("Name"=w331) -> ("String"=w330:string)  [unwired: 9 in, 1 out]
                n175 = Unbundle(w329) -> (w326:string[])
                n176 = Match First String(2:w326, 3:w330) -> (0:w325:i32)  [unwired: 1 out]
                n177 = property on="Ring" class="Ring (strict)"("Value"=w325, "Strings []"=w326) -> ()  [unwired: 2 in, 2 out]
                n178 = property on="Ring" class="Ring (strict)"("Visible"=TRUE) -> ()  [unwired: 2 in, 2 out]
                n179 = property on="Slider" class="Slide (strict)"("Visible"=FALSE) -> ()  [unwired: 2 in, 2 out]
              }
              frame "Exposure  **" {
                n180 = Index Array(array=w337, index=2) -> (element=w338:cluster{string[]})
                n181 = call <vilib>:"NT Read String.vi"("Name"=w340) -> ("String"=w339:string)  [unwired: 9 in, 1 out]
                n182 = Unbundle(w338) -> (w334:string[])
                n183 = Match First String(2:w334, 3:w339) -> (0:w335:i32)  [unwired: 1 out]
                n184 = property on="Ring" class="Ring (strict)"("Value"=w335, "Strings []"=w334) -> ()  [unwired: 2 in, 2 out]
                n185 = property on="Ring" class="Ring (strict)"("Visible"=TRUE) -> ()  [unwired: 2 in, 2 out]
                n186 = property on="Slider" class="Slide (strict)"("Visible"=FALSE) -> ()  [unwired: 2 in, 2 out]
              }
              frame "Exposure Priority  **" {
                n187 = Index Array(array=w346, index=3) -> (element=w347:cluster{string[]})
                n188 = call <vilib>:"NT Read String.vi"("Name"=w349) -> ("String"=w348:string)  [unwired: 9 in, 1 out]
                n189 = Unbundle(w347) -> (w343:string[])
                n190 = Match First String(2:w343, 3:w348) -> (0:w344:i32)  [unwired: 1 out]
                n191 = property on="Ring" class="Ring (strict)"("Value"=w344, "Strings []"=w343) -> ()  [unwired: 2 in, 2 out]
                n192 = property on="Ring" class="Ring (strict)"("Visible"=TRUE) -> ()  [unwired: 2 in, 2 out]
                n193 = property on="Slider" class="Slide (strict)"("Visible"=FALSE) -> ()  [unwired: 2 in, 2 out]
              }
              frame "Color Enable  **" {
                n194 = Index Array(array=w355, index=4) -> (element=w356:cluster{string[]})
                n195 = call <vilib>:"NT Read String.vi"("Name"=w358) -> ("String"=w357:string)  [unwired: 9 in, 1 out]
                n196 = Unbundle(w356) -> (w352:string[])
                n197 = Match First String(2:w352, 3:w357) -> (0:w353:i32)  [unwired: 1 out]
                n198 = property on="Ring" class="Ring (strict)"("Value"=w353, "Strings []"=w352) -> ()  [unwired: 2 in, 2 out]
                n199 = property on="Ring" class="Ring (strict)"("Visible"=TRUE) -> ()  [unwired: 2 in, 2 out]
                n200 = property on="Slider" class="Slide (strict)"("Visible"=FALSE) -> ()  [unwired: 2 in, 2 out]
              }
              frame Default {
                n201 = property on="Ring" class="Ring (strict)"("Visible"=FALSE) -> ()  [unwired: 2 in, 2 out]
                n202 = property on="Slider" class="Slide (strict)"("Visible"=FALSE) -> ()  [unwired: 2 in, 2 out]
              }
              frame "Brightness  **", "Color Level  **", "Compression  **", "FPS  **", "Sharpness  **" {
                n203 = call <vilib>:"NT Read Number.vi"("Name"=w364) -> ("Numeric"=w363:dbl)  [unwired: 9 in, 1 out]
                n204 = local write "Slider"(w363) -> ()
                n205 = property on="Slider" class="Slide (strict)"("Visible"=TRUE, "Scale.Maximum"=100.0 ("Scale.Range:Maximum")) -> ()  [unwired: 2 in, 2 out]
                n206 = property on="Ring" class="Ring (strict)"("Visible"=FALSE) -> ()  [unwired: 2 in, 2 out]
              }
            }
          }
        }
        n207 = property on="Progress" class="Clust (strict)"("Visible"=FALSE) -> ()  [unwired: 2 in, 2 out]
      }
      event "Test Name": Mouse Enter {
        # "Populate the ring with the list of tests"
        n208 = event-data() -> ()  [unwired: 1 in, 1 out]
        n209 = call <vilib>:"NT Read String Array.vi"("Name"="TestMode/TestList") -> ("String Array"=w371:string[])  [unwired: 9 in, 1 out]
        n210 = Build Array (concatenate)("Select the test to run...", w371) -> (w370:string[])
        n211 = property on="Test Name" class="Ring (strict)"("Strings []"=w370) -> ()  [unwired: 2 in, 2 out]
      }
      event "Test Name": Value Change {
        w373 = FALSE ("Visible")
        # "Tell the robot the test name to run"
        n212 = event-data() -> ("NewVal"=w377:u16)  [unwired: 1 in]
        n213 = property on="Test Name" class="Ring (strict)"() -> ("Strings []"=w378:string[])  [unwired: 2 in, 2 out]
        n214 = local write "Progress"(T4 {"Test Progress"=0, "Test Progress Text"=""} ("Progress")) -> ()
        n215 = Index Array(array=w378, index=w377) -> (element=w376:string)
        n216 = call <vilib>:"NT Write String.vi"("String"=w376, "Name"="TestMode/TestName") -> ()  [unwired: 9 in, 1 out]
        n217 = property on="Progress" class="Clust (strict)"("Visible"=TRUE) -> ()  [unwired: 2 in, 2 out]
        n218 = property on="Motor" class="Clust (strict)"("Visible"=w373) -> ()  [unwired: 2 in, 2 out]
        n219 = property on="Slider" class="Slide (strict)"("Visible"=w373) -> ()  [unwired: 2 in, 2 out]
        n220 = property on="On/Off" class="Bool (strict)"("Visible"=w373) -> ()  [unwired: 2 in, 2 out]
        n221 = property on="Rev/Fwd" class="Clust (strict)"("Visible"=w373) -> ()  [unwired: 2 in, 2 out]
        n222 = property on="Ring" class="Ring (strict)"("Visible"=w373) -> ()  [unwired: 2 in, 2 out]
      }
      event "Listbox": Double Click {
        n223 = event-data() -> ("PlatMods.Shift"=w381:bool, "Row"=w383:i32)  [unwired: 1 in]
        n224 = case shown="False" w381 {
          tunnel: w383 -> [w387 _]
          tunnel: 1 -> [w386 _]
          frame False {
            n225 = property on="Listbox" class="LstBox (strict)"() -> ("Item Symbols"=w385:i32[])  [unwired: 2 in, 2 out]
            n226 = Replace Array Subset(array=w385, new element=w386, index=w387) -> (w384:i32[])
            n227 = property on="Listbox" class="LstBox (strict)"("Item Symbols"=w384) -> ()  [unwired: 2 in, 2 out]
          }
          frame True {
            w388 = 0 ("Top Row")
            n228 = property on="Listbox" class="LstBox (strict)"() -> ("Number of Rows"=w390:u32)  [unwired: 2 in, 2 out]
            n229 = Initialize Array(0, w390) -> (w389:i32[])
            n230 = property on="Listbox" class="LstBox (strict)"("Top Row"=w388, "Value"=w388, "Item Symbols"=w389) -> ()  [unwired: 2 in, 2 out]
          }
        }
      }
      event "Listbox": Key Down {
        n231 = event-data() -> ("VKey"=w394:T24)  [unwired: 1 in]
        n232 = case shown="\"Left\", \"Right\"" w394 {
          selector: w394 -> [w399 _]
          tunnel: eventvkey."Left" ("VKey") -> [w397 _]
          frame "Left", "Right" {
            n233 = Equal?(x=w397, y=w399) -> (x = y?=w398:bool)
            n234 = Select(t=0, s=w398, f=1) -> (s? t:f=w400:i32)
            n235 = property on="Listbox" class="LstBox (strict)"() -> ("Item Symbols"=w403:i32[])  [unwired: 2 in, 2 out]
            n236 = Replace Array Subset(array=w403, new element=w400, index="Listbox") -> (w402:i32[])
            n237 = property on="Listbox" class="LstBox (strict)"("Item Symbols"=w402) -> ()  [unwired: 2 in, 2 out]
          }
          frame Default {
          }
        }
      }
      event "DB Camera Config": Value Change {
        n238 = event-data() -> ("NewVal"=w407:bool)  [unwired: 1 in]
        n239 = case shown="False" w407 {
          tunnel: w406 -> [w416 _]
          tunnel: [w409 w427] -> w405
          tunnel: w404 -> [w408 w427]
          frame False {
            w423 = "Camera"
            w426 = FALSE ("Visible")
            n240 = local read "Camera Settings"() -> (w415:T1)
            n241 = Index Array(array=w416) -> (element=w419:cluster{string[]})  [unwired: 1 in]
            n242 = Unbundle(w415) -> ("Frate Rate"=w414:i32, "Compression"=w413:i32, "Size"=w417:u16)
            n243 = Unbundle(w419) -> (w418:string[])
            n244 = Index Array(array=w418, index=w417) -> (element=w412:string)
            n245 = call-poly <vilib>:"Write Key.vi"("section"=w423, "value"=w412, "key"="Size", "refnum"=w408) -> ("refnum out"=w425:T23)  [unwired: 2 in, 5 out]
            n246 = call-poly <vilib>:"Write Key.vi"("section"=w423, "value"=w414, "key"="FrameRate", "refnum"=w425) -> ("refnum out"=w424:T23)  [unwired: 1 in, 6 out]
            n247 = property on="Camera Settings" class="Clust (strict)"("Visible"=w426) -> ()  [unwired: 2 in, 2 out]
            n248 = local write "DB Camera Config"(w426) -> ()
            n249 = call-poly <vilib>:"Write Key.vi"("section"=w423, "value"=w413, "key"="Compression", "refnum"=w424) -> ("refnum out"=w410:T23)  [unwired: 1 in, 6 out]
            n250 = call <vilib>:"Close Config Data.vi"("refnum"=w410) -> ("file path"=w411:path)  [unwired: 2 in, 8 out]
            n251 = call <vilib>:"Open Config Data.vi"("configuration file path"=w411) -> ("refnum"=w409:T23)  [unwired: 8 in, 2 out]
          }
          frame True {
            n252 = property on="Camera Settings" class="Clust (strict)"("Visible"=TRUE) -> ()  [unwired: 2 in, 2 out]
          }
        }
      }
      event "Camera Settings": Value Change {
        n253 = event-data() -> ("NewVal"=w440:T1)  [unwired: 1 in]
        n254 = Index Array(array=w436) -> (element=w435:cluster{string[]})  [unwired: 1 in]
        n255 = Unbundle(w440) -> ("Frate Rate"=w431:i32, "Compression"=w430:i32, "Size"=w433:u16)
        n256 = Unbundle(w435) -> (w434:string[])
        n257 = Index Array(array=w434, index=w433) -> (element=w432:string)
        n258 = Format Into String(format string="%s   %dfps   %d%%", w432, w431, w430) -> (resulting string=w437:string)  [unwired: 2 in, 1 out]
        n259 = Build Array(w437) -> (w438:string[])
        n260 = property on="DB Camera Config" class="Bool (strict)"("Strings [4]"=w438) -> ()  [unwired: 2 in, 2 out]
      }
      event "Motor.Enable": Value Change {
        n261 = event-data() -> ("NewVal"=w446:bool)  [unwired: 1 in]
        n262 = Unbundle("Motor") -> ("Value"=w445:dbl)  [unwired: 1 out]
        n263 = Select(t=w445, s=w446, f=0.0) -> (s? t:f=w443:dbl)
        n264 = call <vilib>:"NT Write Number.vi"("Numeric"=w443, "Name"=w442) -> ()  [unwired: 9 in, 1 out]
      }
      event "Slider": Value Change {
        n265 = event-data() -> ("NewVal"=w449:dbl)  [unwired: 1 in]
        n266 = call <vilib>:"NT Write Number.vi"("Numeric"=w449, "Name"=w450) -> ()  [unwired: 9 in, 1 out]
      }
      event "On/Off": Value Change {
        n267 = event-data() -> ("NewVal"=w454:bool)  [unwired: 1 in]
        n268 = Boolean To (0,1)(Boolean=w454) -> (0, 1=w453:i16)
        n269 = call <vilib>:"NT Write Number.vi"("Numeric"=w453, "Name"=w452) -> ()  [unwired: 9 in, 1 out]
      }
      event "Rev/Fwd": Value Change {
        n270 = event-data() -> ("NewVal.Forward"=w462:bool, "NewVal.Reverse"=w461:bool)  [unwired: 1 in]
        n271 = Boolean To (0,1)(Boolean=w462) -> (0, 1=w458:i16)
        n272 = Boolean To (0,1)(Boolean=w461) -> (0, 1=w460:i16)
        n273 = Negate(x=w460) -> (-x=w459:i16)
        n274 = Add(x=w458, y=w459) -> (x+y=w457:i16)
        n275 = call <vilib>:"NT Write Number.vi"("Numeric"=w457, "Name"=w456) -> ()  [unwired: 9 in, 1 out]
      }
      event "Ring": Value Change {
        n276 = event-data() -> ("NewVal"=w466:u16)  [unwired: 1 in]
        n277 = property on="Ring" class="Ring (strict)"() -> ("Strings []"=w467:string[])  [unwired: 2 in, 2 out]
        n278 = Index Array(array=w467, index=w466) -> (element=w465:string)
        n279 = call <vilib>:"NT Write String.vi"("String"=w465, "Name"=w464) -> ()  [unwired: 9 in, 1 out]
      }
    }
  }
  n280 = Index Array(array=w18) -> (element=w19:cluster{string[]})  [unwired: 1 in]
  n281 = Unbundle(w19) -> (w17:string[])
  n282 = Match First String(2:w17, 3:w16) -> (0:w15:i32)  [unwired: 1 out]
  n283 = Bundle("value"=w21, "value"=w20, "index"=w15) -> (w9:cluster{"value":i32, "value":i32, "index":i32})  [unwired: 1 out]
  n284 = property on="On/Off" class="Bool (strict)"("Visible"=w32) -> ()  [unwired: 2 in, 2 out]
  n285 = property on="Motor" class="Clust (strict)"("Visible"=w32) -> ()  [unwired: 2 in, 2 out]
  n286 = property on="Progress" class="Clust (strict)"("Visible"=w32) -> ()  [unwired: 2 in, 2 out]
  n287 = property on="Ring" class="Ring (strict)"("Visible"=w32) -> ()  [unwired: 2 in, 2 out]
  n288 = property on="Camera Settings" class="Clust (strict)"("Val(Sgnl)"=w9) -> ()  [unwired: 2 in, 2 out]
  n289 = property on="Rev/Fwd" class="Clust (strict)"("Visible"=w32) -> ()  [unwired: 2 in, 2 out]
  n290 = property on="Camera Settings" class="Clust (strict)"("Visible"=w32) -> ()  [unwired: 2 in, 2 out]
  n291 = local write "DB Camera Config"(w32) -> ()
